vi "Configure Active Trace.vi"(5 "Format":T1, 7 "S parameter":T2(ring), 8 "error in (no error)":errorcluster, 10 "Active Trace":u8=1, 11 "VNA-ENA in":refnum<class "VNA-ENA.lvclass">) -> (0 "error out":errorcluster, 3 "VNA-ENA out":refnum<class "VNA-ENA.lvclass">)   [LabVIEW 2020, in "VNA-ENA.lvclass"]
doc: "Configures the active trace.\nIt creates the trace and sets the S paramert and mode."
uses:
  VNA-ENA.lvclass
  C:/Sandbox/Git_Sandbox/WiSpry Test Framework source code (LV20)/WiSpry Test Framework/Instruments/Instrument.lvclass
  C:/Sandbox/Git_Sandbox/WiSpry Test Framework source code (LV20)/WiSpry Test Framework/Instruments/Vector Network Analyzer/Vector Network Analyzer.lvclass
  Controls/S parm format enum.ctl
  Instrument.lvclass/Instrument.ctl
  Vector Network Analyzer.lvclass/Vector Network Analyzer.ctl
  Instrument.lvclass
  Vector Network Analyzer.lvclass
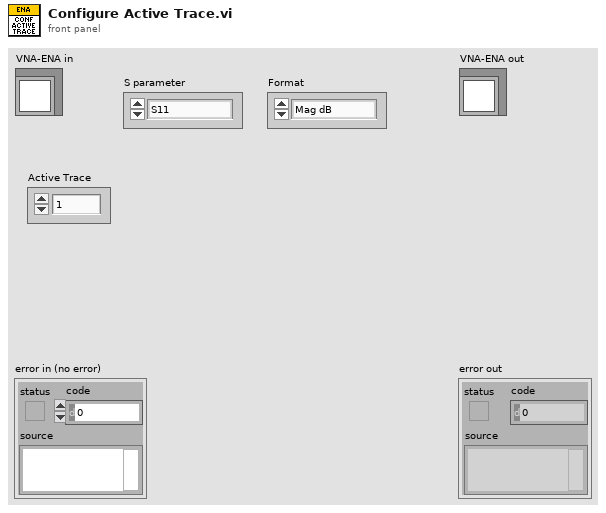
[diagram p1: front panel]
types:
  T1 = typedef "Vector Network Analyzer.lvclass/S parm format enum.ctl" = enum16{"Mag dB", "Mag", "Phase", "Smith", "Real", "Imag", "Group Delay", "SWR"}
  T2 = enum16{"S11", "S21", "S31", "S41", "S22", "S12", "S32", "S42", "S33", "S13", "S23", "S43", "S44", "S14", "S24", "S34"}
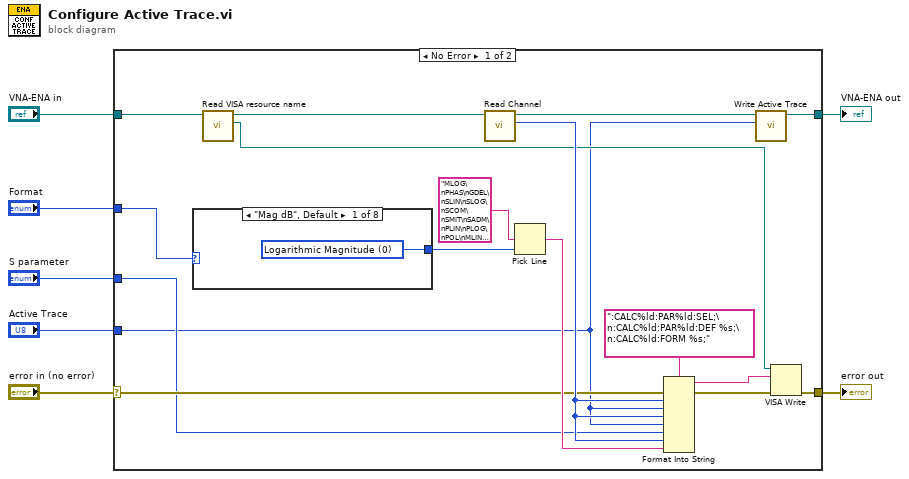
[diagram p0: block diagram]
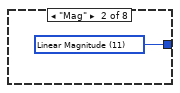
[diagram p2: hidden frame]
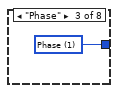
[diagram p3: hidden frame]
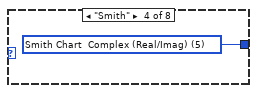
[diagram p4: hidden frame]
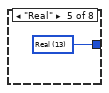
[diagram p5: hidden frame]
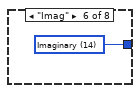
[diagram p6: hidden frame]
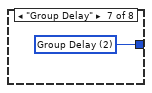
[diagram p7: hidden frame]
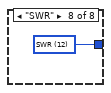
[diagram p8: hidden frame]
diagram:
  n1 = case shown="No Error" "error in (no error)" {
    selector: "error in (no error)" -> [w12 w34]
    tunnel: [w13 w34] -> w7
    tunnel: [w9 w33] -> w6
    tunnel: "Format" -> [w23 _]
    tunnel: "S parameter" -> [w11 _]
    tunnel: "Active Trace" -> [w8 _]
    tunnel: "VNA-ENA in" -> [w24 w33]
    frame No Error {
      n2 = case shown="\"Mag dB\", Default" w23 {
        tunnel: [w25 w26 w27 w28 w29 w30 w31 w32] -> w18
        frame "Mag dB", Default {
          w25 = u16 0 items=["Logarithmic Magnitude", "Phase", "Group Delay", "Smith Chart  Linear (Lin/Phase)", "Smith Chart  Logarithmic (Log/Phase)", "Smith Chart  Complex (Real/Imag)", "Smith Chart  Impedance (R+jX)", "Smith Chart  Admittance (G+jB)", "Polar Format (Linear)", "Polar Format (Logarithmic)", "Polar Format (Re/Im)", "Linear Magnitude", "SWR", "Real", "Imaginary", "Epanded Phase", "Positive Phase"] ("Data Format (0: Logarithmic Magnitude)")
        }
        frame "Mag" {
          w26 = u16 11 items=["Logarithmic Magnitude", "Phase", "Group Delay", "Smith Chart  Linear (Lin/Phase)", "Smith Chart  Logarithmic (Log/Phase)", "Smith Chart  Complex (Real/Imag)", "Smith Chart  Impedance (R+jX)", "Smith Chart  Admittance (G+jB)", "Polar Format (Linear)", "Polar Format (Logarithmic)", "Polar Format (Re/Im)", "Linear Magnitude", "SWR", "Real", "Imaginary", "Epanded Phase", "Positive Phase"] ("Data Format (0: Logarithmic Magnitude)")
        }
        frame "Phase" {
          w27 = u16 1 items=["Logarithmic Magnitude", "Phase", "Group Delay", "Smith Chart  Linear (Lin/Phase)", "Smith Chart  Logarithmic (Log/Phase)", "Smith Chart  Complex (Real/Imag)", "Smith Chart  Impedance (R+jX)", "Smith Chart  Admittance (G+jB)", "Polar Format (Linear)", "Polar Format (Logarithmic)", "Polar Format (Re/Im)", "Linear Magnitude", "SWR", "Real", "Imaginary", "Epanded Phase", "Positive Phase"] ("Data Format (0: Logarithmic Magnitude)")
        }
        frame "Smith" {
          w28 = u16 5 items=["Logarithmic Magnitude", "Phase", "Group Delay", "Smith Chart  Linear (Lin/Phase)", "Smith Chart  Logarithmic (Log/Phase)", "Smith Chart  Complex (Real/Imag)", "Smith Chart  Impedance (R+jX)", "Smith Chart  Admittance (G+jB)", "Polar Format (Linear)", "Polar Format (Logarithmic)", "Polar Format (Re/Im)", "Linear Magnitude", "SWR", "Real", "Imaginary", "Epanded Phase", "Positive Phase"] ("Data Format (0: Logarithmic Magnitude)")
        }
        frame "Real" {
          w29 = u16 13 items=["Logarithmic Magnitude", "Phase", "Group Delay", "Smith Chart  Linear (Lin/Phase)", "Smith Chart  Logarithmic (Log/Phase)", "Smith Chart  Complex (Real/Imag)", "Smith Chart  Impedance (R+jX)", "Smith Chart  Admittance (G+jB)", "Polar Format (Linear)", "Polar Format (Logarithmic)", "Polar Format (Re/Im)", "Linear Magnitude", "SWR", "Real", "Imaginary", "Epanded Phase", "Positive Phase"] ("Data Format (0: Logarithmic Magnitude)")
        }
        frame "Imag" {
          w30 = u16 14 items=["Logarithmic Magnitude", "Phase", "Group Delay", "Smith Chart  Linear (Lin/Phase)", "Smith Chart  Logarithmic (Log/Phase)", "Smith Chart  Complex (Real/Imag)", "Smith Chart  Impedance (R+jX)", "Smith Chart  Admittance (G+jB)", "Polar Format (Linear)", "Polar Format (Logarithmic)", "Polar Format (Re/Im)", "Linear Magnitude", "SWR", "Real", "Imaginary", "Epanded Phase", "Positive Phase"] ("Data Format (0: Logarithmic Magnitude)")
        }
        frame "Group Delay" {
          w31 = u16 2 items=["Logarithmic Magnitude", "Phase", "Group Delay", "Smith Chart  Linear (Lin/Phase)", "Smith Chart  Logarithmic (Log/Phase)", "Smith Chart  Complex (Real/Imag)", "Smith Chart  Impedance (R+jX)", "Smith Chart  Admittance (G+jB)", "Polar Format (Linear)", "Polar Format (Logarithmic)", "Polar Format (Re/Im)", "Linear Magnitude", "SWR", "Real", "Imaginary", "Epanded Phase", "Positive Phase"] ("Data Format (0: Logarithmic Magnitude)")
        }
        frame "SWR" {
          w32 = u16 12 items=["Logarithmic Magnitude", "Phase", "Group Delay", "Smith Chart  Linear (Lin/Phase)", "Smith Chart  Logarithmic (Log/Phase)", "Smith Chart  Complex (Real/Imag)", "Smith Chart  Impedance (R+jX)", "Smith Chart  Admittance (G+jB)", "Polar Format (Linear)", "Polar Format (Logarithmic)", "Polar Format (Re/Im)", "Linear Magnitude", "SWR", "Real", "Imaginary", "Epanded Phase", "Positive Phase"] ("Data Format (0: Logarithmic Magnitude)")
        }
      }
      n3 = call "Read VISA resource name.vi"("Instrument in"=w24) -> ("VISA resource name"=w16:refnum<visa-resource-name>, "Instrument out"=w22:refnum<class "VNA-ENA.lvclass">)  [unwired: 9 in]
      n4 = call-dynamic "Read Channel.vi"("Vector Network Analyzer in"=w22) -> ("Channel"=w20:i32, "Vector Network Analyzer out"=w10:refnum<class "VNA-ENA.lvclass">)  [unwired: 9 in]
      n5 = Pick Line(multi-line string="MLOG\nPHAS\nGDEL\nSLIN\nSLOG\nSCOM\nSMIT\nSADM\nPLIN\nPLOG\nPOL\nMLIN\nSWR\nREAL\nIMAG\nUPH\nPPH" ("string (\"\")"), line index=w18) -> (output string=w17:string)  [unwired: 1 in]
      n6 = Format Into String(format string=":CALC%ld:PAR%ld:SEL;\n:CALC%ld:PAR%ld:DEF %s;\n:CALC%ld:FORM %s;", error in=w12, w20, w8, w20, w8, w11, w20, w17) -> (resulting string=w15:string, error out=w14:errorcluster)  [unwired: 1 in]
      n7 = call "Write Active Trace.vi"("Active Trace"=w8, "Vector Network Analyzer in"=w10) -> ("Vector Network Analyzer out"=w9:refnum<class "VNA-ENA.lvclass">)  [unwired: 9 in]
      n8 = VISA Write(VISA resource name=w16, write buffer=w15, error in (no error)=w14) -> (error out=w13:errorcluster)  [unwired: 2 out]
    }
    frame Error {
    }
  }
  "error out" <- w7
  "VNA-ENA out" <- w6
